vi "Timestamp to Military Time.vi"(11 "Time Stamp":timestamp) -> (3 "Military Time String":string)   [LabVIEW 2018, in "File IO.lvlib"]
doc: "Takes timestamp and converts to military time with no date."
uses:
  File IO.lvlib
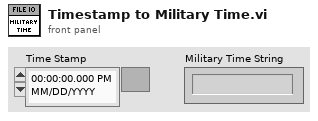
[diagram p1: front panel]
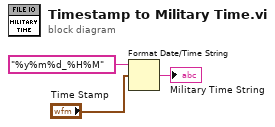
[diagram p0: block diagram]
diagram:
  n1 = Format Date/Time String(time format string (%c)="%y%m%d_%H%M", seconds (now)="Time Stamp") -> (date/time string=→"Military Time String":string)  [unwired: 1 in]
